vi "Get Current Index.vi"(8 "error in (no error)":errorcluster, 11 "PPT in":refnum<class "PPT.lvclass">) -> (0 "error out":errorcluster, 2 "ID":i32, 3 "PPT out":refnum<class "PPT.lvclass">)   [LabVIEW 2014]
uses:
  PPT.lvclass
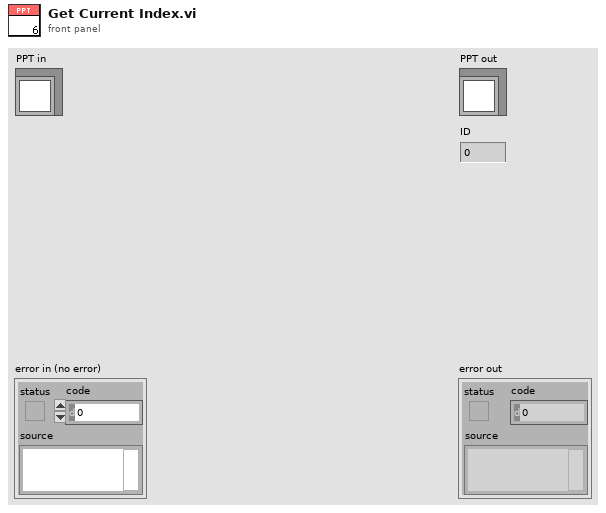
[diagram p1: front panel]
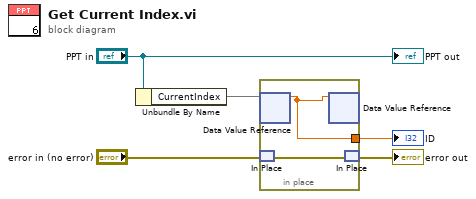
[diagram p0: block diagram]
diagram:
  n1 = Unbundle By Name("PPT in") -> ("CurrentIndex"=w4)
  n2 = in-place {
    in-place-border: [w6] -> w3
    n3 = in-place-dvr #1(w4) -> (w6:dbl)  [unwired: 1 out]
    n4 = in-place-match #2("error in (no error)") -> (w7:errorcluster)
    n5 = in-place-dvr #1(w6) -> ()  [unwired: 2 out]
    n6 = in-place-match #2(w7) -> (→"error out":errorcluster)
  }
  "ID" <- w3
  "PPT out" <- "PPT in"
